vi "Set Processes Queues Map.vi"(8 "Error In":errorcluster, 10 "Processes Queues Map":map{string, refnum<queue>}(c390), 11 "Central Message Handler In":refnum<class "Central Message Handler.lvclass">) -> (0 "Error Out":errorcluster, 3 "Central Message Handler Out":refnum<class "Central Message Handler.lvclass">)   [LabVIEW 2019, in "Central Message Handler.lvclass"]
uses:
  Central Message Handler.lvclass
  Process/Public/Controls/Process Message.ctl
  Process/Process.lvclass
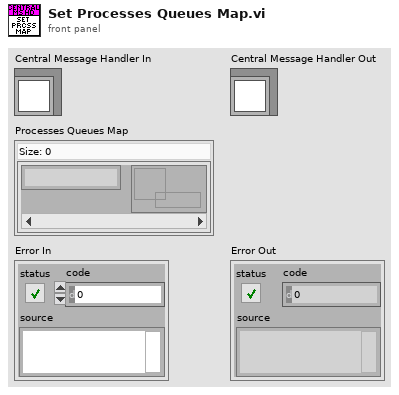
[diagram p1: front panel]
types:
  T1 = typedef "Central Message Handler.lvclass/Data.ctl" = cluster{"Central Message Queue":refnum<queue>, "Processes Queues Map":map{string, refnum<queue>}}
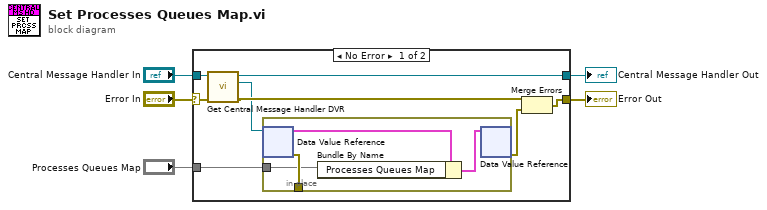
[diagram p0: block diagram]
diagram:
  n1 = case shown="No Error" "Error In" {
    selector: "Error In" -> [w10 w18]
    tunnel: [w12 w18] -> w2
    tunnel: [w9 w19] -> w5
    tunnel: "Central Message Handler In" -> [w11 w19]
    tunnel: "Processes Queues Map" -> [w6 _]
    frame No Error {
      n2 = call "Get Central Message Handler DVR.vi"("Error In"=w10, "Central Message Handler In"=w11) -> ("Error Out"=w8:errorcluster, "DVR"=w7:refnum<data-value>, "Central Message Handler Out"=w9:refnum<class "Central Message Handler.lvclass">)  [unwired: 7 in]
      n3 = in-place {
        in-place-border: [w17] -> _
        in-place-border: w6 -> [w14]
        n4 = in-place-dvr #1(w7) -> (w16:T1, w17:errorcluster)
        n5 = Bundle By Name(cluster=w16, "Processes Queues Map"=w14) -> (w15:T1)
        n6 = in-place-dvr #1(w15) -> (w13:errorcluster)  [unwired: 1 out]
      }
      n7 = Merge Errors(w8, w13) -> (w12:errorcluster)
    }
    frame Error {
    }
  }
  "Central Message Handler Out" <- w5
  "Error Out" <- w2
